vi "Read Callback.vi"(8 "error in (no error)":errorcluster, 11 "Callback in":refnum<class "Callback.lvclass">) -> (0 "error out":errorcluster, 2 "Callback":refnum<vi>, 3 "Callback out":refnum<class "Callback.lvclass">)   [LabVIEW 2017, in "Promise Future.lvlib" / "Callback.lvclass"]
uses:
  Callback.lvclass
  Callback.lvclass/Callback.ctl
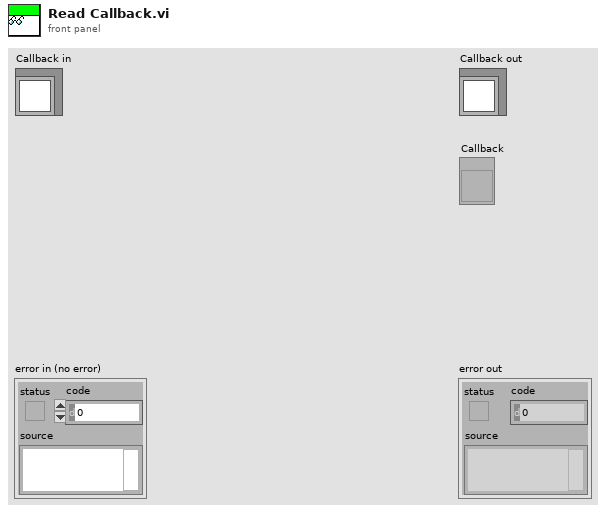
[diagram p1: front panel]
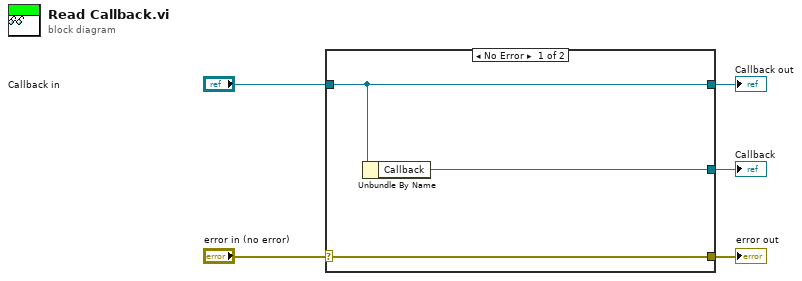
[diagram p0: block diagram]
diagram:
  n1 = case shown="No Error" "error in (no error)" {
    selector: "error in (no error)" -> [w8 w9]
    tunnel: [w8 w9] -> w4
    tunnel: [w7 w10] -> w2
    tunnel: "Callback in" -> [w7 w10]
    tunnel: [w6 _] -> w1
    frame No Error {
      n2 = Unbundle By Name(w7) -> ("Callback"=w6:refnum<vi>)
    }
    frame Error {
    }
  }
  "error out" <- w4
  "Callback out" <- w2
  "Callback" <- w1
